vi "2_Sin(x)(Inference).vi"() -> ()   [LabVIEW 2020]
uses:
  <vilib>/Ngene/Deep Learning Toolkit/Toolkit/NN_Network/Controls/NN_Save_Before_Destroy_Options.ctl
  <vilib>/Ngene/Deep Learning Toolkit/Toolkit/NN_Network/API/NN_Set_Input/1D/NN_Set_Input(1D_SGL_idx).vi
  <vilib>/Ngene/Deep Learning Toolkit/Toolkit/Deep_Learning_Toolkit_by_Ngene.lvlib
panel:
  out "Absalute Error Precentage":sgl=0.004982114 format="%#_2g%%"
  out "sin(x) Predicted":sgl=-0.70978177
  out "sin(x) Ground Truth":sgl=-0.70479965
  in  "Stop":bool
  in  "Weight File Path":path=path "D:/1_Simple_Examples/14_Non-Linear_Regression_Single_Output/working/Sin(x)/Sin(x)_weights_23_08_21__14_23_09.bin"
  in  "CFG File Path":path=path "D:/1_Simple_Examples/14_Non-Linear_Regression_Single_Output/working/Sin(x)/Sin(x)_net_cfg_23_08_21__14_23_09.cfg"
  in  "Input (radians)":sgl(slide)=18.067415 scale=0.0..30.0
  # "Overview: Demonstrates the usage of DeepLTK (Deep Learning Toolkit for LabVIEW) for solving a simple regression problem of modeling sin(x) function.\nRequirements: DeepLTK - Deep Learning Toolkit for LabVIEW (https://www.ngene.co/deep-learning-toolkit-for-labview)\n\nInstructions:\n1. Provide Network Configuration File Path and Weight File Path generated from \"1_Simple_Regression_Sin(x)(Train).vi\".\n2. Run the VI.\n3. Provide input values at Input (radians) control and observe predicted values for sin(x) at sin(x) Predicted and compare it with sin(x) Ground Truth. \n4. Press the Stop button to stop the VI.\n\nMore Examples:  https://github.com/ngenehub/deepltk_examples"
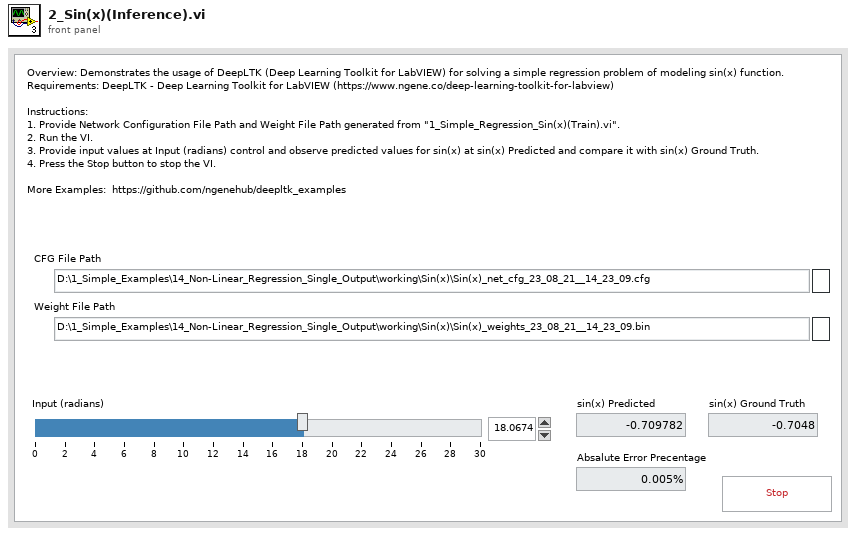
[diagram p1: front panel]
types:
  T1 = typedef "Deep_Learning_Toolkit_by_Ngene.lvlib/NN_Save_Before_Destroy_Options.ctl" = cluster{"CFG?":bool, "Weights?":bool, "Render?":bool}
  T2 = typedef "Deep_Learning_Toolkit_by_Ngene.lvlib/NN_Config_Params.ctl" = cluster{"Name":string, "mBatch":i32, "NN_Train_Params":T3, "LR_Decay_Policy":T6, "Labels":string[], "Loss":T8, "Max_WS_Size(B)":i64, "DryRun?":bool}
  T3 = typedef "Deep_Learning_Toolkit_by_Ngene.lvlib/NN_Train_Params.ctl" = cluster{"Optimizer":T4, "Beta_1":sgl, "Beta_2":sgl, "Weight Decay(L1)":sgl, "Weight Decay(L2)":sgl, "Data_Sampling":T5}
  T4 = typedef "Deep_Learning_Toolkit_by_Ngene.lvlib/NN_Train_Optimizer.ctl" = enum16{"SGD", "Adam", "Adagrad", "Adadelta", "RMSProp", "Nesterov"}
  T5 = typedef "Deep_Learning_Toolkit_by_Ngene.lvlib/NN_Train_Data_Sampling.ctl" = enum16{"Random", "Sequential"}
  T6 = typedef "Deep_Learning_Toolkit_by_Ngene.lvlib/NN_LR_Policy_Cfg.ctl" = cluster{"Policy_Type":T7, "LR0":dbl, "k":sgl, "WarmUp_Policy":enum16{"Step", "Ramp"}, "WarmUp_Iter":i32, "WarmUp_Ratio":sgl}
  T7 = typedef "Deep_Learning_Toolkit_by_Ngene.lvlib/NN_LR_Policy_Type.ctl" = enum16{"Manual", "Step", "Exp", "1/t"}
  T8 = typedef "Deep_Learning_Toolkit_by_Ngene.lvlib/NN_Loss_Config_Params.ctl" = cluster{"Loss_Type":T9, "Loss_Conf_Params":variant}
  T9 = typedef "Deep_Learning_Toolkit_by_Ngene.lvlib/NN_Loss_Type.ctl" = enum16{"None", "MSE", "CrossEntropy", "YOLO_v2", "YOLO_v4"}
  T10 = typedef "Deep_Learning_Toolkit_by_Ngene.lvlib/NN_Layer_Config_Params.ctl" = cluster{"Layer_Type":T11, "Layer_Conf_Params":variant, "Input Layers":string[]}
  T11 = typedef "Deep_Learning_Toolkit_by_Ngene.lvlib/NN_Layer_Type.ctl" = enum16{"Input1D", "Input3D", "Conv1D", "Conv2D", "Conv2D_Adv", "MaxPool", "AvgPool", "UpSample", "DropOut3D", "ShortCut", "Concat", "SoftMax3D", "FC", "DropOut", "Softmax", "Flatten", "YOLO_v2", "YOLO_v4", "Activation", "BatchNormalization", "LayerNormalization", "Scale", "Unsupported"}
  T12 = typedef "Deep_Learning_Toolkit_by_Ngene.lvlib/NN.ctl" = cluster{"Name":string, "No of Layers":i32, "mBatch":i32, "Layers":T13[], "Dimty":T14, "Dims_In":T15, "Dims_Out":T15, "Working_Dir":path, "Train?":bool, "Train_Params":T3, "LR_Update_Policy":T6, "Session Data":T16, "Ground_truth":T17, "NNg_hdls":T18, "NN_Device":T19, "GPU Id":i32, "Labels":string[], "Loss_Type":T9, "Loss_Cfg_Prms":variant, "NNG_WS":T20, "DryRun?":bool}
  T13 = typedef "Deep_Learning_Toolkit_by_Ngene.lvlib/NN_Layer_ref.ctl" = refnum<file>
  T14 = typedef "Deep_Learning_Toolkit_by_Ngene.lvlib/NN_In_Out_Dim-ty.ctl" = enum8{"In1D_Out1D", "In3D_Out1D", "In3D_Out3D", "In3D_OutBBox"}
  T15 = typedef "Deep_Learning_Toolkit_by_Ngene.lvlib/NN_Dims(C,H,W).ctl" = cluster{"C":i32, "H":i32, "W":i32}
  T16 = typedef "Deep_Learning_Toolkit_by_Ngene.lvlib/NN_Train_Session_Data.ctl" = cluster{"Epochs":sgl, "Tot_Iter":i32, "LR":sgl, "LR_iter":i32}
  T17 = typedef "Deep_Learning_Toolkit_by_Ngene.lvlib/NN_Ground_truth.ctl" = cluster{"Y":variant}
  T18 = typedef "Deep_Learning_Toolkit_by_Ngene.lvlib/nng_cuda_handles.ctl" = cluster{"cudnn":u64, "cublas":u64, "stream":u64, "curand":u64}
  T19 = typedef "Deep_Learning_Toolkit_by_Ngene.lvlib/NN_Device.ctl" = enum16{"CPU", "GPU"}
  T20 = typedef "Deep_Learning_Toolkit_by_Ngene.lvlib/NNG_WS.ctl" = cluster{"NNG_WS_Mem":T21, "Max_WS_Size":i64}
  T21 = typedef "Deep_Learning_Toolkit_by_Ngene.lvlib/NNg_WS_Mem_DVR.ctl" = refnum<data-value>
  T22 = typedef "Deep_Learning_Toolkit_by_Ngene.lvlib/NN_Layer.ctl" = cluster{"Name":string, "Layer_Data":T23, "Layer_Type":T11, "Dims_In":T15, "Layers_In":T13[], "Dims_Out":T15, "Layers_Out":T13[], "Metrics":T24, "GPU_Data":T25, "mBatch":i32, "NN_Device":T19, "NNg_hdls":T18, "Train?":bool, "Dimty":T26, "RecptField":T27, "Idx":i32}
  T23 = typedef "Deep_Learning_Toolkit_by_Ngene.lvlib/NN_Layer_Data_Refnum.ctl" = refnum<file>
  T24 = typedef "Deep_Learning_Toolkit_by_Ngene.lvlib/NN_Layer_Metrics.ctl" = cluster{"Data":dbl, "Params":dbl, "Ops":dbl}
  T25 = typedef "Deep_Learning_Toolkit_by_Ngene.lvlib/NNg_Layer_Data_Refnum.ctl" = refnum<file>
  T26 = typedef "Deep_Learning_Toolkit_by_Ngene.lvlib/NN_Layer_Dimty.ctl" = enum16{"1D", "3D"}
  T27 = typedef "Deep_Learning_Toolkit_by_Ngene.lvlib/NN_Layer_RF_State.ctl" = cluster{"Dims":T28, "J":T28}
  T28 = typedef "Deep_Learning_Toolkit_by_Ngene.lvlib/NN_Dims(V,H).ctl" = cluster{"V":i32, "H":i32}
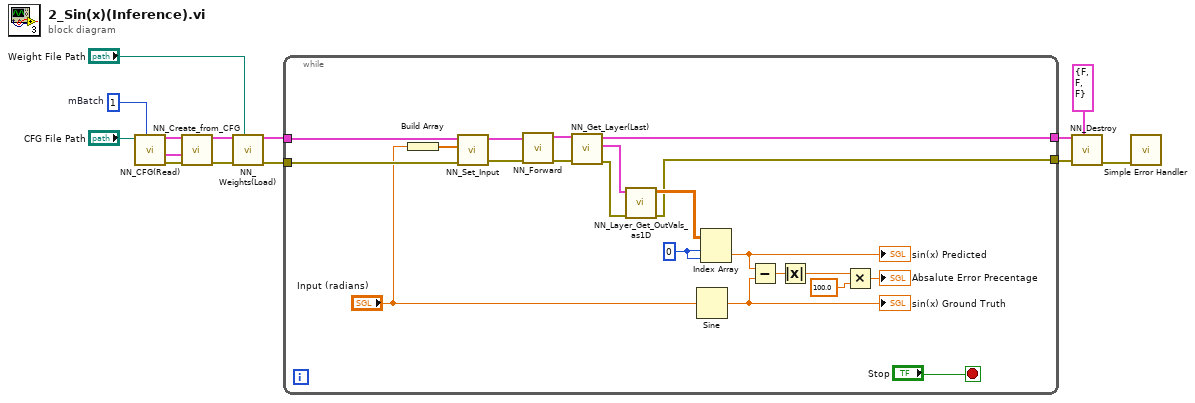
[diagram p0: block diagram]
diagram:
  w5 = 1  # mBatch
  n1 = call <vilib>:"NN_CFG(Read).vi"("mBatch"=w5, "CFG file path"="CFG File Path") -> ("error out"=w14:errorcluster, "Net_Cfg"=w6:T2, "Layer_Cfg"=w11:T10[])  [unwired: 7 in]
  n2 = call <vilib>:"NN_Create_from_CFG.vi"("error in (no error)"=w14, "Net_Cfg"=w6, "Layer_Cfg"=w11) -> ("error out"=w13:errorcluster, "NN out"=w12:T12)  [unwired: 7 in]
  n3 = call <vilib>:"NN_Weights(Load).vi"("Weight File Path"="Weight File Path", "error in (no error)"=w13, "NN in"=w12) -> ("error out"=w9:errorcluster, "NN out"=w10:T12)  [unwired: 7 in]
  n4 = while {
    tunnel: w10 -> [w34]
    tunnel: w9 -> [w35]
    tunnel: [w27] -> w8
    tunnel: [w23] -> w7
    stop <- "Stop" stop-if-true
    w25 = 0 ("disabled index (col)")
    n5 = Build Array("Input (radians)") -> (w24:sgl[])
    n6 = call-poly <vilib>:"NN_Set_Input.vi"("error in (no error)"=w35, "Data_In(1D_SGL)"=w24, "NN In"=w34) -> ("error out"=w32:errorcluster, "NN Out"=w33:T12)  [unwired: 7 in]
    n7 = call <vilib>:"NN_Forward.vi"("error in (no error)"=w32, "NN in"=w33) -> ("error out"=w31:errorcluster, "NN out"=w30:T12)  [unwired: 6 in, 2 out]
    n8 = call <vilib>:"NN_Get_Layer(Last).vi"("error in (no error)"=w31, "NN in"=w30) -> ("error out"=w29:errorcluster, "Last_Layer"=w28:T22, "NN out"=w27:T12)  [unwired: 6 in, 1 out]
    n9 = call <vilib>:"NN_Layer_Get_OutVals_as1D.vi"("error in (no error)"=w29, "Layer"=w28) -> ("error out"=w23:errorcluster, "Out(as1D)"=w26:sgl[][])  [unwired: 8 in]
    n10 = Sine(x="Input (radians)") -> (sin(x)=w19:sgl)
    "sin(x) Ground Truth" <- w19
    n11 = Index Array(array=w26, index (row)=w25, index (col)=w25) -> (element=w20:sgl)
    "sin(x) Predicted" <- w20
    n12 = Subtract(x=w20, y=w19) -> (x-y=w18:sgl)
    n13 = Absolute Value(x=w18) -> (abs(x)=w17:sgl)
    n14 = Multiply(x=w17, y=sgl 100.0) -> (x*y=→"Absalute Error Precentage":sgl)
  }
  n15 = call <vilib>:"NN_Destroy.vi"("Save (T, T, T)"=T1 {"CFG?"=FALSE, "Weights?"=FALSE, "Render?"=FALSE}, "error in (no error)"=w7, "NN in"=w8) -> ("error out"=w1:errorcluster)  [unwired: 7 in, 1 out]
  n16 = call <vilib>:"Simple Error Handler.vi"("error in (no error)"=w1) -> ()  [unwired: 4 in, 5 out]
